vi "Read Roles.vi"(8 "error in (no error)":errorcluster, 11 "BallPlacementPlay in":refnum<class "BallPlacementPlay.lvclass">) -> (0 "error out":errorcluster, 2 "Roles":T1, 3 "BallPlacementPlay out":refnum<class "BallPlacementPlay.lvclass">)   [LabVIEW 2021, in "BallPlacementPlay.lvclass"]
uses:
  BallPlacementPlay.lvclass
  BallPlacementEnemyRole_class/BallPlacementEnemyRole.lvclass
  BallPlacementPlay.lvclass/BallPlacementPlay.ctl
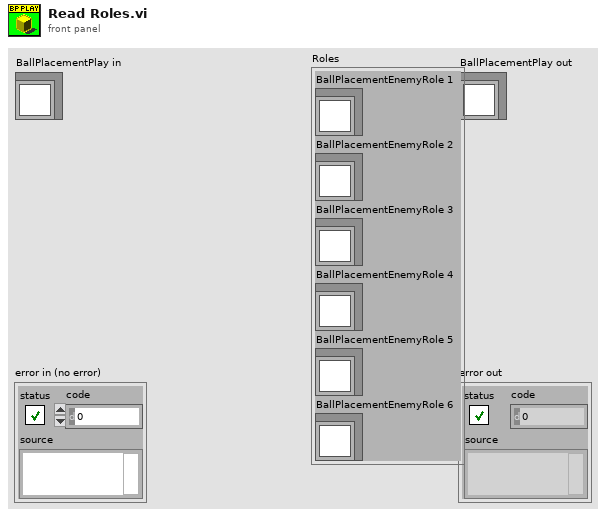
[diagram p1: front panel]
types:
  T1 = cluster{"BallPlacementEnemyRole 1":refnum<class "BallPlacementEnemyRole.lvclass">, "BallPlacementEnemyRole 2":refnum<class "BallPlacementEnemyRole.lvclass">, "BallPlacementEnemyRole 3":refnum<class "BallPlacementEnemyRole.lvclass">, "BallPlacementEnemyRole 4":refnum<class "BallPlacementEnemyRole.lvclass">, "BallPlacementEnemyRole 5":refnum<class "BallPlacementEnemyRole.lvclass">, "BallPlacementEnemyRole 6":refnum<class "BallPlacementEnemyRole.lvclass">}
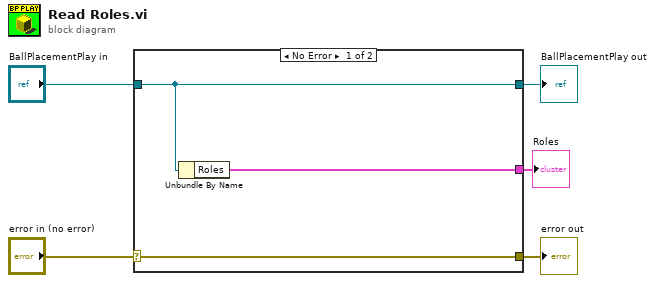
[diagram p0: block diagram]
diagram:
  n1 = case shown="No Error" "error in (no error)" {
    selector: "error in (no error)" -> [w8 w9]
    tunnel: [w8 w9] -> w4
    tunnel: [w7 w10] -> w2
    tunnel: "BallPlacementPlay in" -> [w7 w10]
    tunnel: [w6 _] -> w1
    frame No Error {
      n2 = Unbundle By Name(w7) -> ("Roles"=w6:T1)
    }
    frame Error {
    }
  }
  "error out" <- w4
  "BallPlacementPlay out" <- w2
  "Roles" <- w1
